vi "System_Simulation.vi"() -> ()   [LabVIEW 2014]
uses:
  <vilib>/Simulation/Scripting/Companion Diagram/SimConfigNode/SimParams.ctl
  <vilib>/Simulation/Scripting/Companion Diagram/SimConfigNode/_simSolvers.ctl
  <vilib>/Simulation/Implementation/Shared/SIMSCR Execution Mode.ctl
  <vilib>/Simulation/Param Hierarchy/Typedefs/SIMPH Param Control Actions.ctl
  <vilib>/Simulation/Implementation/Shared/NILVSim_ParamChanged.vi
  <vilib>/Simulation/Implementation/Shared/NILVSIM_BeginStep.vi
  <vilib>/Simulation/DataSources/Implementation/NILVSim Pulse Generator.llb/SIM Pulse Generator (scalar).vi
  <vilib>/Simulation/ContinuousLinear/Implementation/NILVSim Transfer Function.llb/SIM Transfer Function Distributor (SISO).vi
  <vilib>/Simulation/ContinuousLinear/Implementation/NILVSim Transfer Function.llb/SIM Transfer Function Collector (SISO).vi
  <vilib>/Simulation/SignalDisplay/Implementation/NILVSim Time Waveform.llb/SIM Time Waveform (scalar).vi
  <vilib>/Simulation/Implementation/Shared/NILVSim_Manager.vi
  <vilib>/Utility/error.llb/Clear Errors.vi
  <vilib>/Simulation/Implementation/Shared/NILVSim_FinalizeModel.vi
  <vilib>/Simulation/Implementation/Shared/SIM Unbundle Sim Info.vi
  <vilib>/Simulation/Implementation/Shared/NILVSim_Initialize.vi
  <vilib>/ptbypt/Signal Generation.llb/Gaussian White Noise PtByPt.vi
  <vilib>/Simulation/Utility/Implementation/NILVSim Get Time and IsAcceptedStep.vi
  <vilib>/Simulation/Implementation/Shared/SIMSH Read Queue.vi
  <vilib>/Simulation/Implementation/Shared/NILVSim_GetModelError.vi
  <vilib>/Simulation/Implementation/Shared/SIM Bundle Sim Info.vi
  <vilib>/Simulation/Scripting/Companion Diagram/SimConfigNode/SimDog.xnode
  <vilib>/Simulation/Implementation/XNodeFramework/SimXNode/SimX.xnode
  <vilib>/ptbypt/NI_PtbyPt.lvlib
  <vilib>/Simulation/ContinuousLinear/Implementation/NILVSim Transfer Function.llb/SIM Transfer Function (SISO).vi
  <vilib>/Simulation/Implementation/Shared/NI_SIM_Implementation.lvlib
panel:
  out "Phase spectrum":cluster{"f0":dbl, "df":dbl, "phase":dbl[]}(graph)
  out "Amplitude spectrum":cluster{"f0":dbl, "df":dbl, "magnitude":dbl[]}(graph)
  in  "Freq (Hz)":dbl=500000.0
  out "Output":waveform(i16)(graph)={"t0"=timestamp(0 s since 1904-01-01), "dt"=2e-06, "Y"=array[5001 elements]}
  out "Input":waveform(i16)(graph)={"t0"=timestamp(0 s since 1904-01-01), "dt"=2e-06, "Y"=array[5001 elements]}
  out "System ID":waveform(dbl)(graph)={"t0"=timestamp(0 s since 1904-01-01), "dt"=2e-06, "Y"=array[5001 elements]}
  in  "CS_R(ohm)":dbl=500000.0
  in  "INA R(ohm)":dbl=100000.0
  out "Waveform Chart":waveform(dbl)(graph)={"t0"=timestamp(0.01 s since 1904-01-01), "dt"=1.0, "Y"=[1.8810764409104788]}
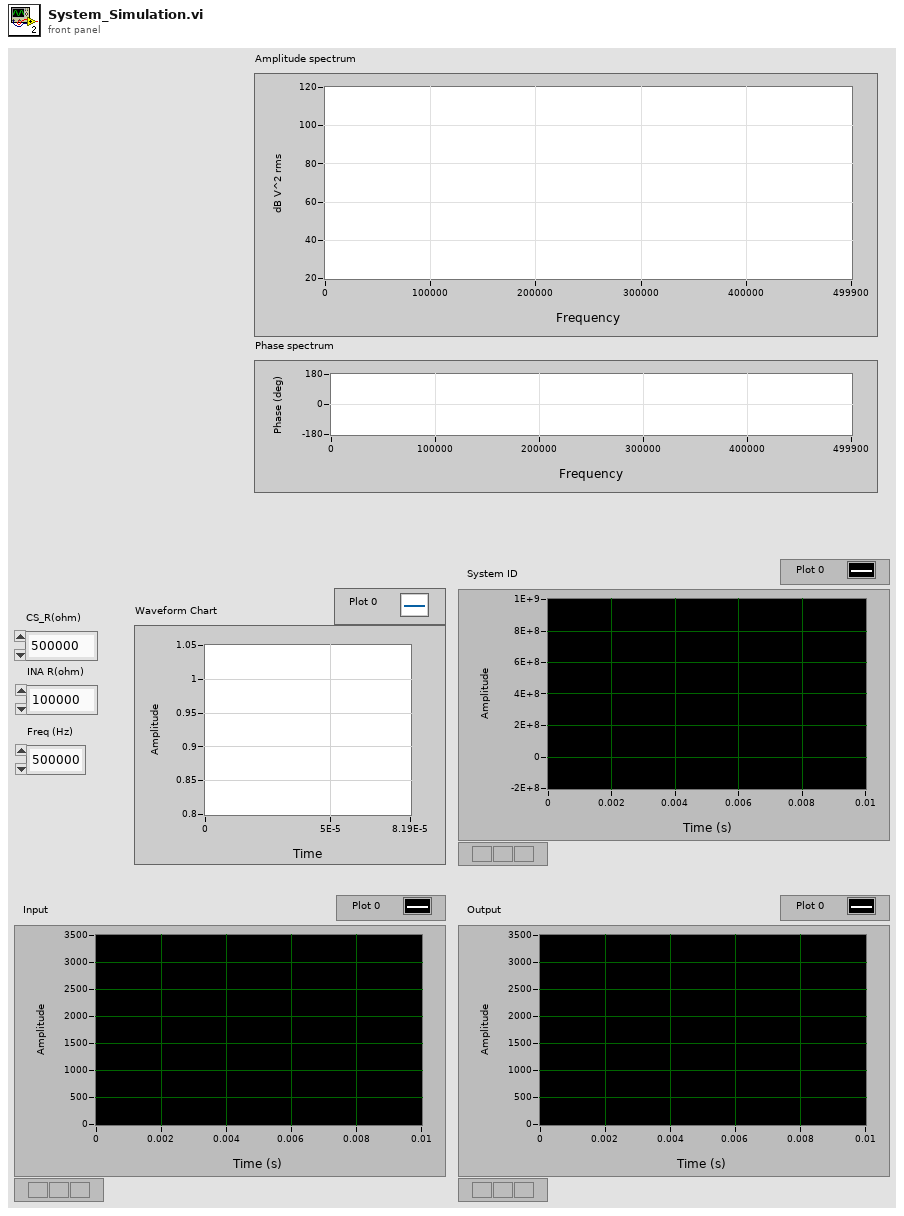
[diagram p1: front panel]
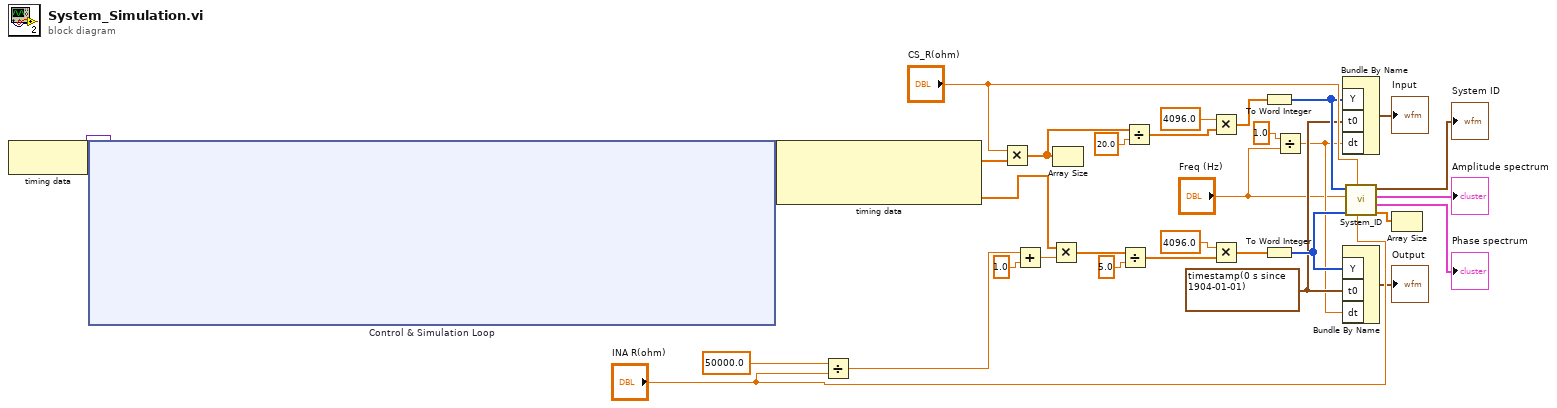
[diagram p0: block diagram]
diagram:
  w6 = timestamp(0 s since 1904-01-01) ("t0")
  n1 = node-c288() -> (w32:variant)  [unwired: 1 in]
  n2 = node-c254 "Control & Simulation Loop"(w32) -> (w31:variant)
  n3 = node-c288(w31) -> (w13:dbl[], w17:dbl[])  [unwired: 1 out]
  n4 = Divide(x=50000.0, y="INA R(ohm)") -> (x/y=w19:dbl)
  n5 = Multiply(x="CS_R(ohm)", y=w13) -> (x*y=w11:dbl[])
  n6 = Add(x=w19, y=1.0 ("x")) -> (x+y=w18:dbl)
  n7 = Multiply(x=w17, y=w18) -> (x*y=w26:dbl[])
  n8 = Array Size(array=w11) -> ()  [unwired: 1 out]
  n9 = Divide(x=w26, y=5.0 ("f")) -> (x/y=w24:dbl[])
  n10 = Divide(x=w11, y=20.0 ("f")) -> (x/y=w29:dbl[])
  n11 = Multiply(x=4096.0 ("f"), y=w29) -> (x*y=w27:dbl[])
  n12 = Multiply(x=4096.0 ("f"), y=w24) -> (x*y=w22:dbl[])
  n13 = To Word Integer(number=w27) -> (16bit integer=w10:i16[])
  n14 = To Word Integer(number=w22) -> (16bit integer=w7:i16[])
  n15 = Divide(x=1.0, y="Freq (Hz)") -> (x/y=w5:dbl)
  n16 = Bundle By Name("Y"=w10, "t0"=w6, "dt"=w5) -> (→"Input":waveform(i16))  [unwired: 1 in]
  n17 = Bundle By Name("Y"=w7, "t0"=w6, "dt"=w5) -> (→"Output":waveform(i16))  [unwired: 1 in]
  n18 = call "System_ID.vi"("INA Resistance (ohm)"="INA R(ohm)", "Current Source Resistance (ohm)"="CS_R(ohm)", "Input Y"=w7, "Sample_Frequency (Hz)"="Freq (Hz)", "Input X"=w10) -> ("x*y"=w12:dbl[], "Phase spectrum"=→"Phase spectrum":cluster{"f0":dbl, "df":dbl, "phase":dbl[]}, "Amplitude spectrum"=→"Amplitude spectrum":cluster{"f0":dbl, "df":dbl, "magnitude":dbl[]}, "Actuation Graph"=→"System ID":waveform(dbl))  [unwired: 3 in]
  n19 = Array Size(array=w12) -> ()  [unwired: 1 out]
